vi "Get Array Values as Numerics.vi"(8 "error in (no error)":errorcluster, 11 "JSON Array in":refnum<class "JSON Helper.lvclass">) -> (0 "error out":errorcluster, 3 "values":dbl[](array[numeric]))   [LabVIEW 2016, in "JSON Helper.lvclass"]
doc: "Returns the element type of each element in a JSON Array. If all elements are of the same type, single type is true."
uses:
  JSON Helper/JSON Helper.lvclass
  JSON Types.ctl
  Errors/Errors.ctl
  JSON Numeric/Read value (Numeric).vi
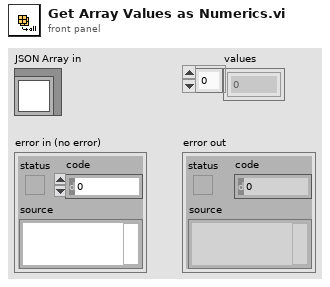
[diagram p1: front panel]
types:
  T1 = typedef "JSON Helper.lvclass/JSON Types.ctl" = enum16{"String", "Numeric", "Boolean", "NULL", "Object", "Array"}
  T2 = typedef "JSON Helper.lvclass/Errors.ctl" = enum16{"No key", "Key path type", "Array OOB", "Type Mismatch", "Invalid Token"}
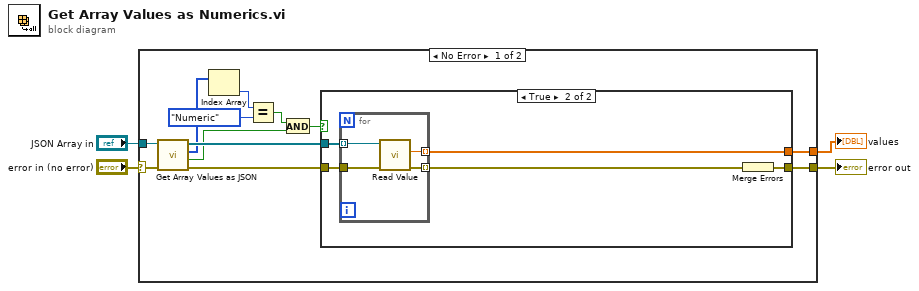
[diagram p0: block diagram]
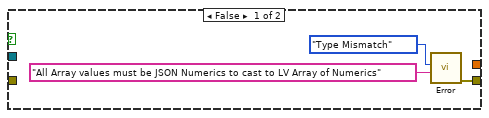
[diagram p2: hidden frame]
diagram:
  n1 = case shown="No Error" "error in (no error)" {
    selector: "error in (no error)" -> [w15 w29]
    tunnel: "JSON Array in" -> [w16 _]
    tunnel: [w13 w29] -> w2
    tunnel: [w6 _] -> w1
    frame No Error {
      n2 = call "Get Array Values as JSON.vi"("error in (no error)"=w15, "JSON Array in"=w16) -> ("error out"=w5:errorcluster, "single type?"=w8:bool, "types"=w12:T1[], "values"=w14:refnum<class "JSON Helper.lvclass">[])  [unwired: 6 in]
      n3 = Index Array(array=w12) -> (element=w11:T1)  [unwired: 1 in]
      n4 = Equal?(x=w11, y=JSON_Types."Numeric") -> (x = y?=w9:bool)
      n5 = And(x=w9, y=w8) -> (x .and. y?=w7:bool)
      n6 = case shown="True" w7 {
        tunnel: w14 -> [_ w24]
        tunnel: [w17 w20] -> w13
        tunnel: [_ w23] -> w6
        tunnel: w5 -> [_ w21]
        frame False {
          n7 = call "Error.vi"("Data"="All Array values must be JSON Numerics to cast to LV Array of Numerics", 9:Errors."Type Mismatch") -> ("error out"=w17:errorcluster)  [unwired: 8 in]
        }
        frame True {
          n8 = for {
            tunnel: w24 -> [w25] mode=indexing
            tunnel: [w28] -> w23 mode=indexing
            tunnel: [w27] -> w22 mode=indexing
            tunnel: w21 -> [w26]
            n9 = call-poly "Read Value.vi"("error in (no error)"=w26, "JSON Numeric in"=w25) -> ("error out"=w27:errorcluster, "value"=w28:dbl)  [unwired: 8 in]
          }
          n10 = Merge Errors(w22) -> (w20:errorcluster)
        }
      }
    }
    frame Error {
    }
  }
  "error out" <- w2
  "values" <- w1
